vi "Talker.vi"(0 "Divide in":refnum<class "Divide.lvclass">, 5 "Subpanel Ref":refnum<vi>, 11 "Error In":errorcluster) -> (4 "Divide out":refnum<class "Divide.lvclass">, 15 "Error Out":errorcluster)   [LabVIEW 2020, in "Divide.lvclass"]
uses:
  Divide.lvclass
  Divide.lvclass/Divide.ctl
  UI.vi
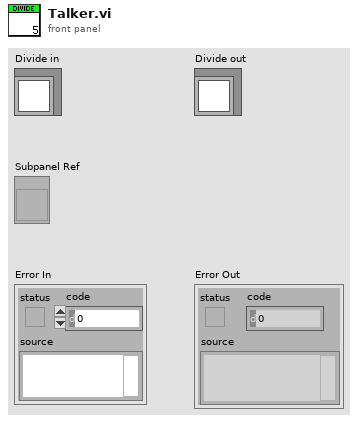
[diagram p1: front panel]
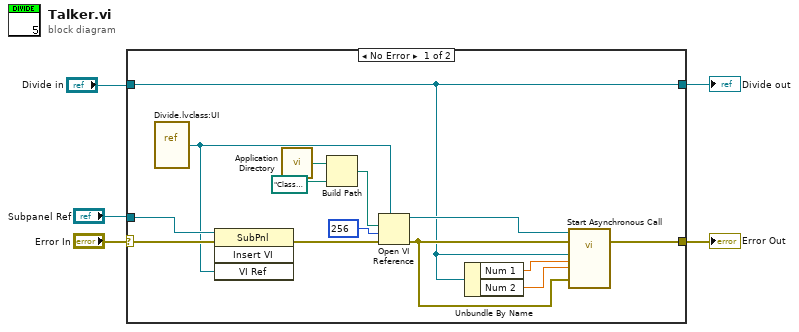
[diagram p0: block diagram]
diagram:
  n1 = case shown="No Error" "Error In" {
    selector: "Error In" -> [w14 w21]
    tunnel: [w7 w21] -> w4
    tunnel: [w8 w20] -> w2
    tunnel: "Divide in" -> [w8 w20]
    tunnel: "Subpanel Ref" -> [w12 _]
    frame No Error {
      n2 = vi-ref "Divide.lvclass:UI.vi"() -> (w6:refnum<vi>)
      n3 = invoke on="Invoke Node" class="SubPnl" method="Insert VI"(reference=w12, error in=w14, "VI Ref"=w6) -> (error out=w13:errorcluster)  [unwired: 1 in, 3 out]
      n4 = call <vilib>:"Application Directory.vi"() -> ("Application Directory"=w15:path)
      n5 = Build Path(base path=w15, name or relative path=path "Classes/Children/Divide/Methods/UI.vi") -> (appended path=w10:path)
      n6 = Open VI Reference(type specifier VI Refnum (for type only)=w6, vi path=w10, options=256, error in (no error)=w13) -> (vi reference=w11:refnum<vi>, error out=w17:errorcluster)  [unwired: 2 in]
      n7 = Unbundle By Name(w8) -> ("Num 1"=w19:dbl, "Num 2"=w18:dbl)
      n8 = call-by-ref "Start Asynchronous Call"(reference=w11, error in=w17, "Divide in"=w8, "Num 1"=w19, "Num 2"=w18, "Error In"=w17) -> (error out=w7:errorcluster)  [unwired: 9 in, 4 out]
    }
    frame Error {
    }
  }
  "Divide out" <- w2
  "Error Out" <- w4
